vi "test_SetEnabledState_SetEnabled_EventLogged.vi"(8 "error in (no error)":errorcluster, 11 "TestCase in":refnum<class "TestDataSink.lvclass">) -> (0 "error out":errorcluster, 3 "TestCase out":refnum<class "TestDataSink.lvclass">)   [LabVIEW 2017, in "TestDataSink.lvclass"]
uses:
  TestDataSink.lvclass
  Source/Composed Log/Types/Log Level.ctl
  Source/LVQueue Sink/LVQueue Sink.lvclass/LVQueue Sink.ctl
  Source/Composed Log/LoggerReference/LoggerReference.lvclass/LoggerReference.ctl
  Source/Composed Log/Log Sink/Log Sink.lvclass/Log Sink.ctl
  e8a6295c-8cd0-4cda-8693-0aa66d3e646b.vi
  e8a6295c-8cd0-4cda-8693-0aa66d3e646b.vi/92e9ac20-7810-47de-9f69-b5a4c855bad2.vi
  Source/Composed Log/LoggerReference/Return Aggregate Queues.vi
  Source/Composed Log/LoggerReference/Add Aggregate Log.vi
  e8a6295c-8cd0-4cda-8693-0aa66d3e646b.vi/92e9ac20-7810-47de-9f69-b5a4c855bad2.vi/bc622e31-8f52-44b4-b9c5-4b59e2be6b1e.vi
  Source/Composed Log/LoggerReference/Log.vi
  Source/Composed Log/LoggerReference/Send Add Sink.vi
  Source/Composed Log/LoggerReference/Remove Stale Logs.vi
  Source/LVQueue Sink/LVQueue Sink.lvclass
  C:/CS/Internal/LabVIEW/Logger/Source/Composed Log/Log Sink/Log Sink.lvclass
  Source/Composed Log/Application Logger/Launch Worker Loop.vi
  Source/Composed Log/LoggerReference/Initialize Logger Instance.vi
  Source/Composed Log/Singleton Event Log/Logger Queue FGV.vi
  Source/Composed Log/IErrorFormat/IErrorFormat.lvclass
  Source/Composed Log/LoggerReference/LoggerReference.lvclass
  Source/Composed Log/Log Sink/Log Sink.lvclass
  Source/Composed Log/Singleton Event Log/Singleton Event Log.lvlib
  Source/Composed Log/Composed Log.lvlib
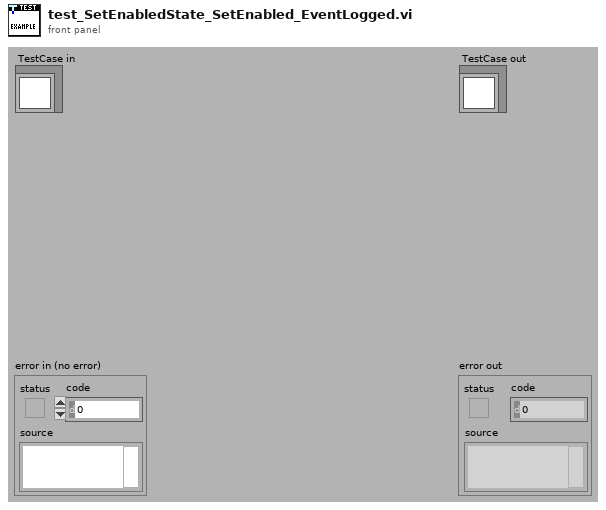
[diagram p1: front panel]
types:
  T1 = typedef "Composed Log.lvlib/Log Level.ctl" = enum16{"Debug", "Info", "Warning", "Error", "Critical"}
  T2 = typedef "Composed Log.lvlib/Log Packet.ctl" = cluster{"Data To Log":string, "Source":string, "Event Level":T1, "Event Time":timestamp}
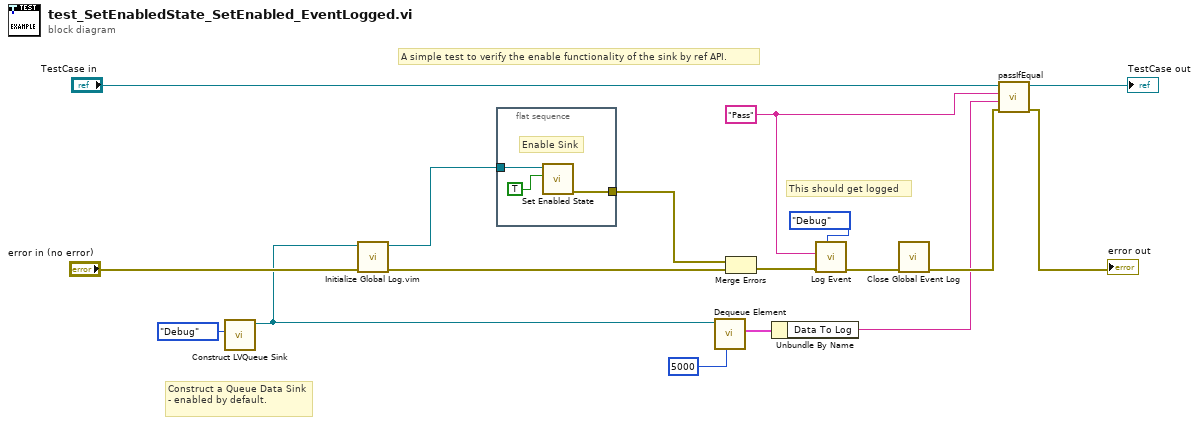
[diagram p0: block diagram]
diagram:
  w3 = "Pass" ("Data To Log")
  # "A simple test to verify the enable functionality of the sink by ref API."
  # "This should get logged"
  # "Construct a Queue Data Sink - enabled by default."
  n1 = call "Construct LVQueue Sink.vi"("LogLevel"=Log_Level."Debug") -> ("LVQueue Sink out"=w6:refnum<class "LVQueue Sink.lvclass">)  [unwired: 9 in, 1 out]
  n2 = call "Initialize Global Log.vim"("error in (no error)"="error in (no error)", "Log Sink(s)"=w6) -> ("error out"=w7:errorcluster, "Log Sink Reference(s)"=w5:refnum<data-value>)  [unwired: 8 in]
  n3 = flat-sequence {
    tunnel: [w19] -> w9
    tunnel: w5 -> [w18]
    frame #0 {
      # "Enable Sink"
      n4 = call "Set Enabled State.vi"("Enabled?"=TRUE, "Log Sink"=w18) -> ("error out"=w19:errorcluster)  [unwired: 9 in]
    }
  }
  n5 = call "Dequeue Element.vi"("timeout in ms (-1)"=5000, "LVQueue Sink in"=w6) -> ("Log Packet"=w10:T2)  [unwired: 6 in, 3 out]
  n6 = Merge Errors(w9, w7) -> (w4:errorcluster)
  n7 = Unbundle By Name(w10) -> ("Data To Log"=w8:string)
  n8 = call "Log Event.vi"("Event Level"=Log_Level."Debug", "error in (no error)"=w4, "Data To Log"=w3) -> ("error out"=w1:errorcluster)  [unwired: 8 in]
  n9 = call "Close Global Event Log.vi"("error in (no error)"=w1) -> ("error out"=w11:errorcluster)  [unwired: 10 in]
  n10 = call-dynamic "passIfEqual.vi"("error in (no error)"=w11, "y"=w8, "x"=w3, "TestCase in"="TestCase in") -> ("error out"=→"error out":errorcluster, "TestCase out"=→"TestCase out":refnum<class "TestDataSink.lvclass">)  [unwired: 6 in]
